vi "Find Next Position of T - Buggy.vi"(1 "Current Position of T":cdb, 3 "Previous Position of H":cdb, 4 "Current Position of H":cdb) -> (5 "Next Position of T":cdb)   [LabVIEW 2020, in "AoC 2022.lvlib"]
uses:
  AoC 2022.lvlib
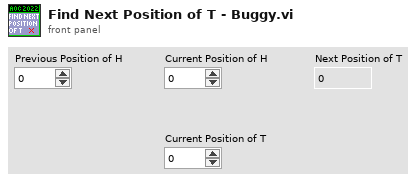
[diagram p1: front panel]
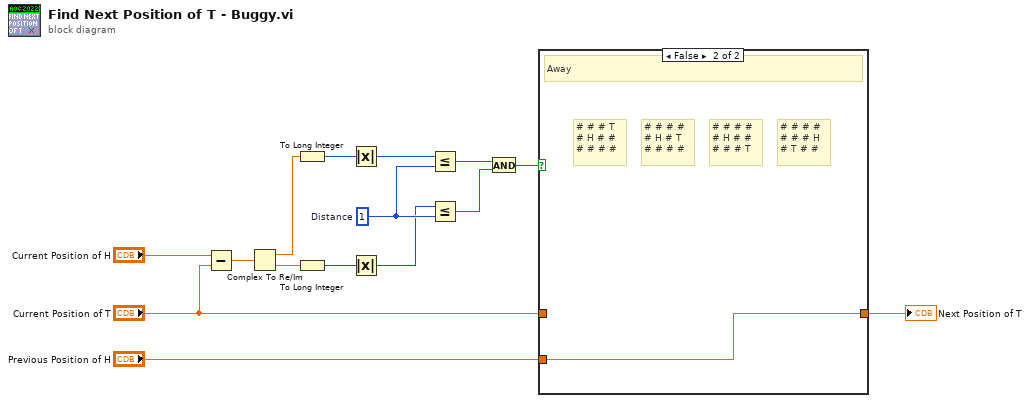
[diagram p0: block diagram]
diagram:
  w9 = 1  # Distance
  n1 = Subtract(x="Current Position of H", y="Current Position of T") -> (x-y=w4:cdb)
  n2 = Complex To Re/Im(x + iy=w4) -> (x=w10:dbl, y=w11:dbl)
  n3 = To Long Integer(number=w10) -> (32bit integer=w8:i32)
  n4 = To Long Integer(number=w11) -> (32bit integer=w7:i32)
  n5 = Absolute Value(x=w8) -> (abs(x)=w6:i32)
  n6 = Absolute Value(x=w7) -> (abs(x)=w5:i32)
  n7 = Less Or Equal?(x=w6, y=w9) -> (x <= y?=w3:bool)
  n8 = Less Or Equal?(x=w5, y=w9) -> (x <= y?=w2:bool)
  n9 = And(x=w3, y=w2) -> (x .and. y?=w1:bool)
  n10 = case shown="False" w1 {
    tunnel: [w16 w17] -> w15
    tunnel: "Current Position of T" -> [w16 _]
    tunnel: "Previous Position of H" -> [_ w17]
    frame True {
      # "T # # #\n# H # #\n# # # #"
      # "# # # #\n# H # #\nT # # #"
      # "# # # #\n# H # #\n# # T #"
      # "# # T #\n# H # #\n# # # #"
      # "# # # #\n# H # #\n# T # #"
      # "# T # #\n# H # #\n# # # #"
      # "# # # #\nT H # #\n# # # #"
      # "# # # #\n# H T #\n# # # #"
      # "Adjacent: Still Touching"
    }
    frame False {
      # "# # # #\n# # # H\n# T # #"
      # "# # # #\n# H # T\n# # # #"
      # "# # # #\n# H # #\n# # # T"
      # "# # # T\n# H # #\n# # # #"
      # "Away"
    }
  }
  "Next Position of T" <- w15
